vi "EMB_Debug_Map_RV_Fixed.vi"(2 "error in (no error)":errorcluster, 3 "Generate Integer Only":bool) -> (0 "error out":errorcluster)   [LabVIEW 2011]
uses:
  <vilib>/LabVIEW Targets/Embedded/Debug/DD/utils/EMB_Debug_DD_GetSetAttrib_String.vi
panel:
  in  "SymbolList IntegerOnly":cluster{"Name":string, "Value":string}[](array[cluster])=[{"Name"="_PDAStr", "Value"="12"}, {"Name"="_PDAStr.refcnt", "Value"="0,16"}, {"Name"="_PDAStr.staticStr", "Value"="16,16"}, {"Name"="_PDAStr.len", "Value"="32,32"}, {"Name"="_PDAStr.str", "Value"="64,16"}, {"Name"="NumericData", "Value"="24"}, {"Name"="NumericData.datatype", "Value"="0,32"}, {"Name"="NumericData.datasize", "Value"="32,8"}, {"Name"="NumericData.bStatic", "Value"="40,8"}, {"Name"="NumericData.bInput", "Value"="48,8"}, {"Name"="NumericData.padding1", "Value"="56,8"}, {"Name"="NumericData.pData", "Value"="64,128"}, {"Name"="StringData", "Value"="16"}, {"Name"="StringData.len", "Value"="0,32"}, {"Name"="StringData.bufferLen", "Value"="32,32"}, {"Name"="StringData.bStatic", "Value"="64,8"}, {"Name"="StringData.padding", "Value"="72,24"}, {"Name"="StringData.pValue", "Value"="96,32"}, {"Name"="_ControlData", "Value"="20"}, {"Name"="_ControlData.controlIdx", "Value"="0,32"}, {"Name"="_ControlData.parentIdx", "Value"="32,32"}, {"Name"="_ControlData.hValue", "Value"="64,32"}, {"Name"="_ControlData.dataType", "Value"="96,32"}, {"Name"="_ControlData.fieldType", "Value"="128,32"}, {"Name"="_OCDI_Alignment", "Value"="8"}, {"Name"="_OCDI_Alignment.el_1", "Value"="0,8"}, {"Name"="_OCDI_Alignment.el_2", "Value"="32,32"}, {"Name"="BooleanData", "Value"="4"}, {"Name"="BooleanData.bStatic", "Value"="0,8"}, {"Name"="BooleanData.bVal", "Value"="8,8"}, {"Name"="BooleanData.bInput", "Value"="24,8"}, {"Name"="BooleanData.bDefaultVal", "Value"="16,8"}, {"Name"="_PDAArr", "Value"="16"}, {"Name"="_PDAArr.datatype", "Value"="0,32"}, {"Name"="_PDAArr.refcnt", "Value"="32,16"}, {"Name"="_PDAArr.staticArray", "Value"="48,8"}, {"Name"="_PDAArr.arr", "Value"="64,32"}, {"Name"="_PDAArr.fill", "Value"="56,8"}, {"Name"="_PDAArr.nDimSize", "Value"="8"}, {"Name"="PictInfo", "Value"="52"}, {"Name"="PictInfo.refcnt", "Value"="0,16"}, {"Name"="PictInfo.dirty", "Value"="16,16"}, {"Name"="PictInfo.dc", "Value"="32,32"}, {"Name"="PictInfo.currentX", "Value"="64,32"}, {"Name"="PictInfo.currentY", "Value"="96,32"}, {"Name"="PictInfo.bounds", "Value"="128,64"}, {"Name"="PictInfo.currentForeColor", "Value"="192,32"}, {"Name"="EnumCtlData", "Value"="20"}, {"Name"="EnumCtlData.nValue", "Value"="32,32"}, {"Name"="EnumCtlData.bStatic", "Value"="128,8"}, {"Name"="EnumCtlData.bInput", "Value"="136,8"}, {"Name"="EnumCtlData.numItems", "Value"="96,32"}, {"Name"="EnumCtlData.datatype", "Value"="0,32"}, {"Name"="EnumCtlData.defaultVal", "Value"="64,32"}, {"Name"="_LVGraphData", "Value"="16"}, {"Name"="_LVGraphData.dtDataIn", "Value"="32,32"}, {"Name"="_LVGraphData.bStatic", "Value"="64,8"}, {"Name"="_LVGraphData.datatype", "Value"="0,32"}, {"Name"="_LVGraphData.vhDataIn", "Value"="96,32"}, {"Name"="ArrayControlData", "Value"="24"}, {"Name"="ArrayControlData.bStatic", "Value"="64,8"}, {"Name"="ArrayControlData.dataType", "Value"="160,32"}, {"Name"="ArrayControlData.elt_datatype", "Value"="128,32"}, {"Name"="ArrayControlData.hDefaultValue", "Value"="32,32"}, {"Name"="ArrayControlData.hValue", "Value"="0,32"}, {"Name"="ArrayControlData.nDims", "Value"="96,32"}, {"Name"="ClusterControlData", "Value"="152"}, {"Name"="ClusterControlData.pBigCls", "Value"="96,32"}, {"Name"="ClusterControlData.pDefaultVal", "Value"="32,32"}, {"Name"="ClusterControlData.pOldVal", "Value"="0,32"}, {"Name"="ClusterControlData.pSmallCls", "Value"="128,1024"}, {"Name"="ClusterControlData.pVal", "Value"="64,32"}]
  in  "SymbolList":cluster{"Name":string, "Value":string}[](array[cluster])=[{"Name"="_PDAStr", "Value"="12"}, {"Name"="_PDAStr.refcnt", "Value"="0,16"}, {"Name"="_PDAStr.staticStr", "Value"="16,16"}, {"Name"="_PDAStr.len", "Value"="32,32"}, {"Name"="_PDAStr.str", "Value"="64,16"}, {"Name"="NumericData", "Value"="24"}, {"Name"="NumericData.datatype", "Value"="0,32"}, {"Name"="NumericData.datasize", "Value"="32,8"}, {"Name"="NumericData.bStatic", "Value"="40,8"}, {"Name"="NumericData.bInput", "Value"="48,8"}, {"Name"="NumericData.padding1", "Value"="56,8"}, {"Name"="NumericData.pData", "Value"="64,128"}, {"Name"="StringData", "Value"="16"}, {"Name"="StringData.len", "Value"="0,32"}, {"Name"="StringData.bufferLen", "Value"="32,32"}, {"Name"="StringData.bStatic", "Value"="64,8"}, {"Name"="StringData.padding", "Value"="72,24"}, {"Name"="StringData.pValue", "Value"="96,32"}, {"Name"="_ControlData", "Value"="20"}, {"Name"="_ControlData.controlIdx", "Value"="0,32"}, {"Name"="_ControlData.parentIdx", "Value"="32,32"}, {"Name"="_ControlData.hValue", "Value"="64,32"}, {"Name"="_ControlData.dataType", "Value"="96,32"}, {"Name"="_ControlData.fieldType", "Value"="128,32"}, {"Name"="_OCDI_Alignment", "Value"="16"}, {"Name"="_OCDI_Alignment.el_1", "Value"="0,8"}, {"Name"="_OCDI_Alignment.el_2", "Value"="64,64"}, {"Name"="BooleanData", "Value"="4"}, {"Name"="BooleanData.bStatic", "Value"="0,8"}, {"Name"="BooleanData.bVal", "Value"="8,8"}, {"Name"="BooleanData.bInput", "Value"="24,8"}, {"Name"="BooleanData.bDefaultVal", "Value"="16,8"}, {"Name"="_PDAArr", "Value"="16"}, {"Name"="_PDAArr.datatype", "Value"="0,32"}, {"Name"="_PDAArr.refcnt", "Value"="32,16"}, {"Name"="_PDAArr.staticArray", "Value"="48,8"}, {"Name"="_PDAArr.arr", "Value"="64,32"}, {"Name"="_PDAArr.fill", "Value"="56,8"}, {"Name"="_PDAArr.nDimSize", "Value"="8"}, {"Name"="PictInfo", "Value"="52"}, {"Name"="PictInfo.refcnt", "Value"="0,16"}, {"Name"="PictInfo.dirty", "Value"="16,16"}, {"Name"="PictInfo.dc", "Value"="32,32"}, {"Name"="PictInfo.currentX", "Value"="64,32"}, {"Name"="PictInfo.currentY", "Value"="96,32"}, {"Name"="PictInfo.bounds", "Value"="128,64"}, {"Name"="PictInfo.currentForeColor", "Value"="192,32"}, {"Name"="EnumCtlData", "Value"="20"}, {"Name"="EnumCtlData.nValue", "Value"="32,32"}, {"Name"="EnumCtlData.bStatic", "Value"="128,8"}, {"Name"="EnumCtlData.bInput", "Value"="136,8"}, {"Name"="EnumCtlData.numItems", "Value"="96,32"}, {"Name"="EnumCtlData.datatype", "Value"="0,32"}, {"Name"="EnumCtlData.defaultVal", "Value"="64,32"}, {"Name"="_LVGraphData", "Value"="16"}, {"Name"="_LVGraphData.dtDataIn", "Value"="32,32"}, {"Name"="_LVGraphData.bStatic", "Value"="64,8"}, {"Name"="_LVGraphData.datatype", "Value"="0,32"}, {"Name"="_LVGraphData.vhDataIn", "Value"="96,32"}, {"Name"="ArrayControlData", "Value"="24"}, {"Name"="ArrayControlData.bStatic", "Value"="64,8"}, {"Name"="ArrayControlData.dataType", "Value"="160,32"}, {"Name"="ArrayControlData.elt_datatype", "Value"="128,32"}, {"Name"="ArrayControlData.hDefaultValue", "Value"="32,32"}, {"Name"="ArrayControlData.hValue", "Value"="0,32"}, {"Name"="ArrayControlData.nDims", "Value"="96,32"}, {"Name"="ClusterControlData", "Value"="152"}, {"Name"="ClusterControlData.pBigCls", "Value"="96,32"}, {"Name"="ClusterControlData.pDefaultVal", "Value"="32,32"}, {"Name"="ClusterControlData.pOldVal", "Value"="0,32"}, {"Name"="ClusterControlData.pSmallCls", "Value"="128,1024"}, {"Name"="ClusterControlData.pVal", "Value"="64,32"}]
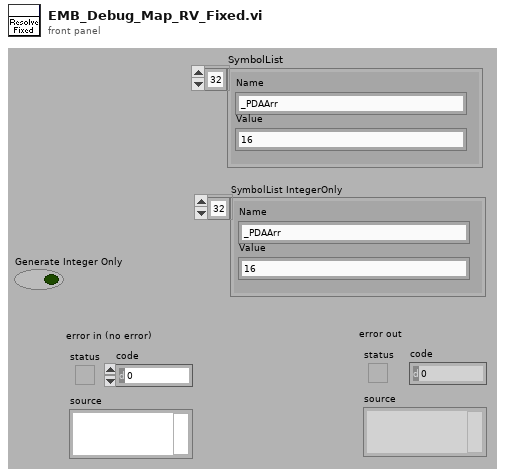
[diagram p1: front panel]
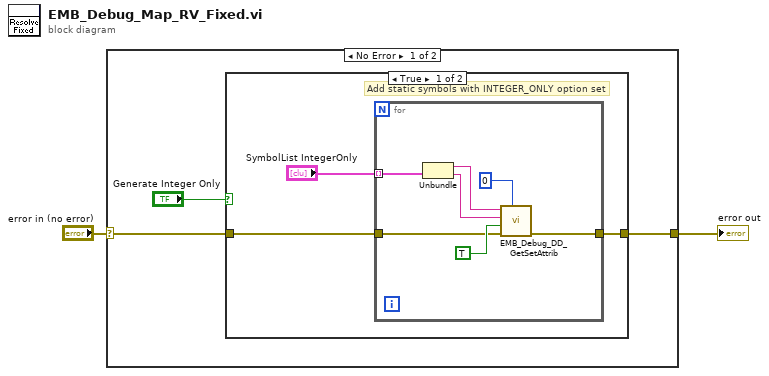
[diagram p0: block diagram]
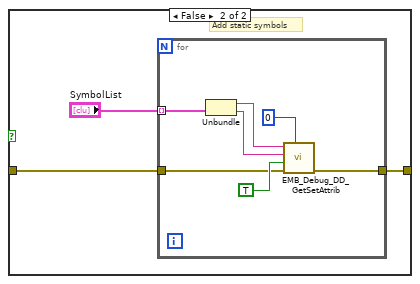
[diagram p2: hidden frame]
diagram:
  n1 = case shown="No Error" "error in (no error)" {
    selector: "error in (no error)" -> [w5 w26]
    tunnel: [w4 w26] -> w1
    frame No Error {
      n2 = case shown="True" "Generate Integer Only" {
        tunnel: w5 -> [w7 w18]
        tunnel: [w6 w16] -> w4
        frame True {
          # "Add static symbols with INTEGER_ONLY option set"
          n3 = for {
            tunnel: w7 -> [w14]
            tunnel: [w13] -> w6
            tunnel: "SymbolList IntegerOnly" -> [w12] mode=indexing
            n4 = Unbundle(w12) -> ("Name"=w11:string, "Value"=w10:string)
            n5 = call-poly <vilib>:"EMB_Debug_DD_GetSetAttrib.vi"("target ID"=u32 0, "error in (no error)"=w14, "set"=TRUE, "value"=w10, "name"=w11) -> ("error out"=w13:errorcluster)  [unwired: 4 in, 2 out]
          }
        }
        frame False {
          # "Add static symbols"
          n6 = for {
            tunnel: w18 -> [w24]
            tunnel: [w23] -> w16
            tunnel: "SymbolList" -> [w22] mode=indexing
            n7 = Unbundle(w22) -> ("Name"=w21:string, "Value"=w20:string)
            n8 = call-poly <vilib>:"EMB_Debug_DD_GetSetAttrib.vi"("target ID"=u32 0, "error in (no error)"=w24, "set"=TRUE, "value"=w20, "name"=w21) -> ("error out"=w23:errorcluster)  [unwired: 4 in, 2 out]
          }
        }
      }
    }
    frame Error {
    }
  }
  "error out" <- w1
